vi "Single String(us) to Stamp.vi"(5 "time string(us)":string) -> (2 "time stamp(us)":timestamp format="%<%.6X\n%x>T")   [LabVIEW 2020]
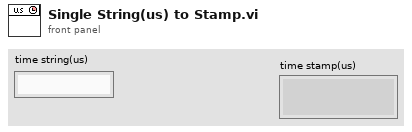
[diagram p1: front panel]
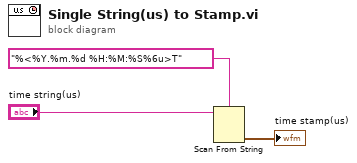
[diagram p0: block diagram]
diagram:
  n1 = Scan From String(format string="%<%Y.%m.%d %H:%M:%S%6u>T", input string="time string(us)") -> (output 1=→"time stamp(us)":timestamp)  [unwired: 3 in, 3 out]
